vi "Get Data Log File Span Settings.vi"(8 "error in":errorcluster, 11 "File Ref In":T1 format="%.0x") -> (0 "error out":errorcluster, 1 "Span by Time":bool, 2 "Maximum Log Time":u32, 3 "File Ref Out":T1 format="%.0x", 4 "Span by Size":bool, 6 "Maximum File Size":u32)   [LabVIEW 2018, in "Embedded Data Logger Shared.lvlib"]
uses:
  <vilib>/NI Veristand/Custom Device API/Custom Device Item Ref.ctl
  Shared/Constants.vi
  <vilib>/NI Veristand/Custom Device API/Get Item Property (U32).vi
  <vilib>/NI Veristand/Custom Device API/Get Item Property (Boolean).vi
  Shared/Embedded Data Logger Shared.lvlib
  <vilib>/NI Veristand/Custom Device API/Custom Device API.lvlib
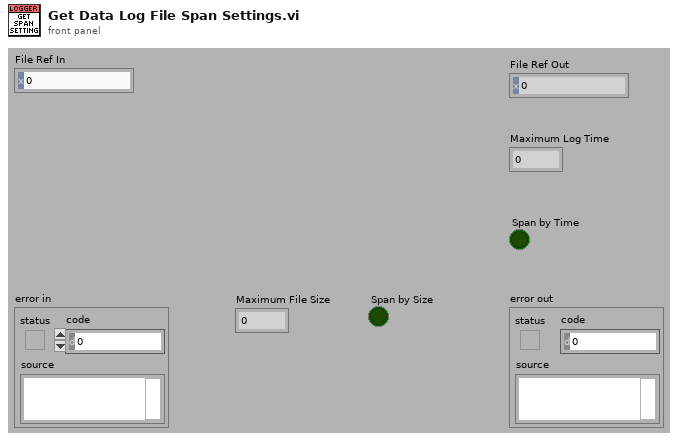
[diagram p1: front panel]
types:
  T1 = typedef "Custom Device API.lvlib/Custom Device Item Ref.ctl" = u64
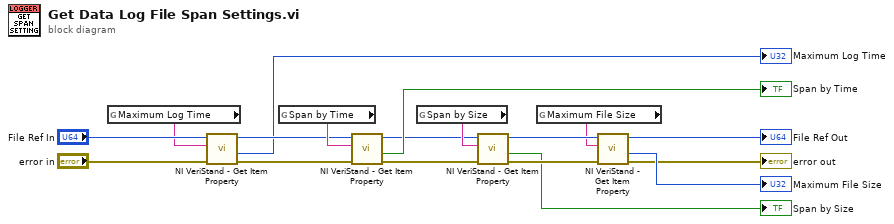
[diagram p0: block diagram]
diagram:
  n1 = global read "Constants.vi" "Maximum Log Time"() -> (w11:string)
  n2 = call-poly <vilib>:"NI VeriStand - Get Item Property.vi"("error in (no error)"="error in", "Property Name"=w11, "Item Ref in"="File Ref In") -> ("error out"=w5:errorcluster, "Value"=→"Maximum Log Time":u32, "Item Ref out"=w6:T1)  [unwired: 1 in, 5 out]
  n3 = global read "Constants.vi" "Span by Time"() -> (w9:string)
  n4 = call-poly <vilib>:"NI VeriStand - Get Item Property.vi"("error in (no error)"=w5, "Property Name"=w9, "Item Ref in"=w6) -> ("error out"=w3:errorcluster, "Value"=→"Span by Time":bool, "Item Ref out"=w4:T1)  [unwired: 1 in, 5 out]
  n5 = global read "Constants.vi" "Span by Size"() -> (w10:string)
  n6 = call-poly <vilib>:"NI VeriStand - Get Item Property.vi"("error in (no error)"=w3, "Property Name"=w10, "Item Ref in"=w4) -> ("error out"=w13:errorcluster, "Value"=→"Span by Size":bool, "Item Ref out"=w14:T1)  [unwired: 1 in, 5 out]
  n7 = global read "Constants.vi" "Maximum File Size"() -> (w2:string)
  n8 = call-poly <vilib>:"NI VeriStand - Get Item Property.vi"("error in (no error)"=w13, "Property Name"=w2, "Item Ref in"=w14) -> ("error out"=→"error out":errorcluster, "Value"=→"Maximum File Size":u32, "Item Ref out"=→"File Ref Out":T1)  [unwired: 1 in, 5 out]
